vi "add overlays.vi"(8 "error in (no error)":errorcluster, 9 "location constraints":T2(array[cluster]), 10 "Overlay Rectangles":T1(array[cluster]), 11 "color ims":cluster{"xy im":T3, "xz im":T3, "zy im":T3}) -> (0 "error out":errorcluster, 3 "color ims out":cluster{"xy im":T3, "xz im":T3, "zy im":T3})   [LabVIEW 2010]
uses:
  <vilib>/vision/Image Controls.llb/IMAQ Image.ctl
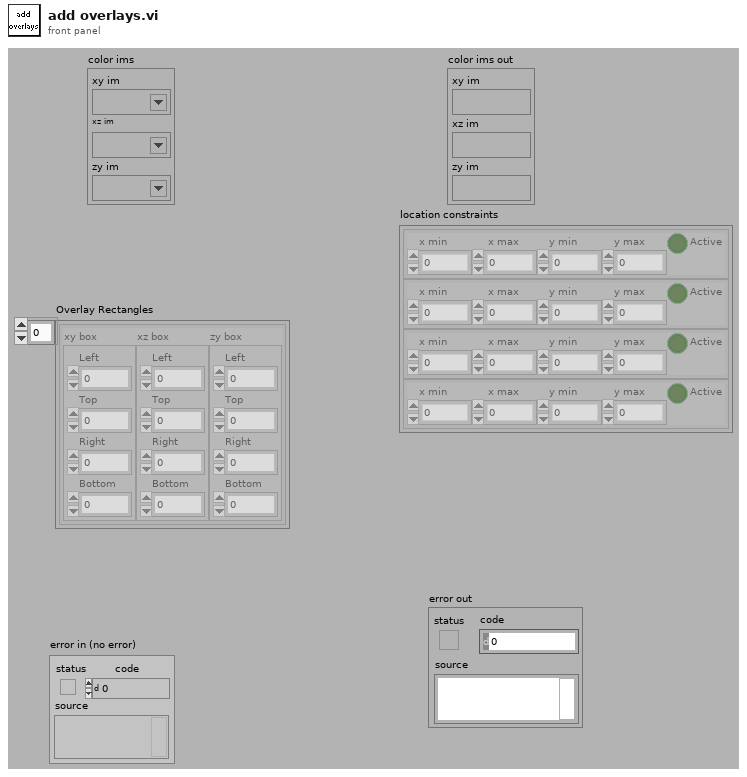
[diagram p1: front panel]
types:
  T1 = cluster{"xy box":cluster{"Left":i32, "Top":i32, "Right":i32, "Bottom":i32}, "xz box":cluster{"Left":i32, "Top":i32, "Right":i32, "Bottom":i32}, "zy box":cluster{"Left":i32, "Top":i32, "Right":i32, "Bottom":i32}}[]
  T2 = cluster{"x min":i32, "x max":i32, "y min":i32, "y max":i32, "Active":bool}[]
  T3 = typedef "IMAQ Image.ctl" = refnum<image>
  T4 = cluster{"Desired Font (Application)":enum16{"User-specified Font", "Application Font", "System Font", "Dialog Font"}, "[User-specified Font]":cluster{"Font Name":string, "Size":i16, "Strikeout?":bool, "Italic?":bool, "Underline?":bool, "Outline?":bool, "Shadow?":bool, "Bold?":bool, "Rotation Angle":dbl}, "Horizontal Alignment":i16, "Vertical Alignment":i16}
  T5 = cluster{"Left":i32, "Top":i32, "Right":i32, "Bottom":i32}
  T6 = cluster{"Left":i32, "Top":i32, "Right":i32, "Bottom":i32}[]
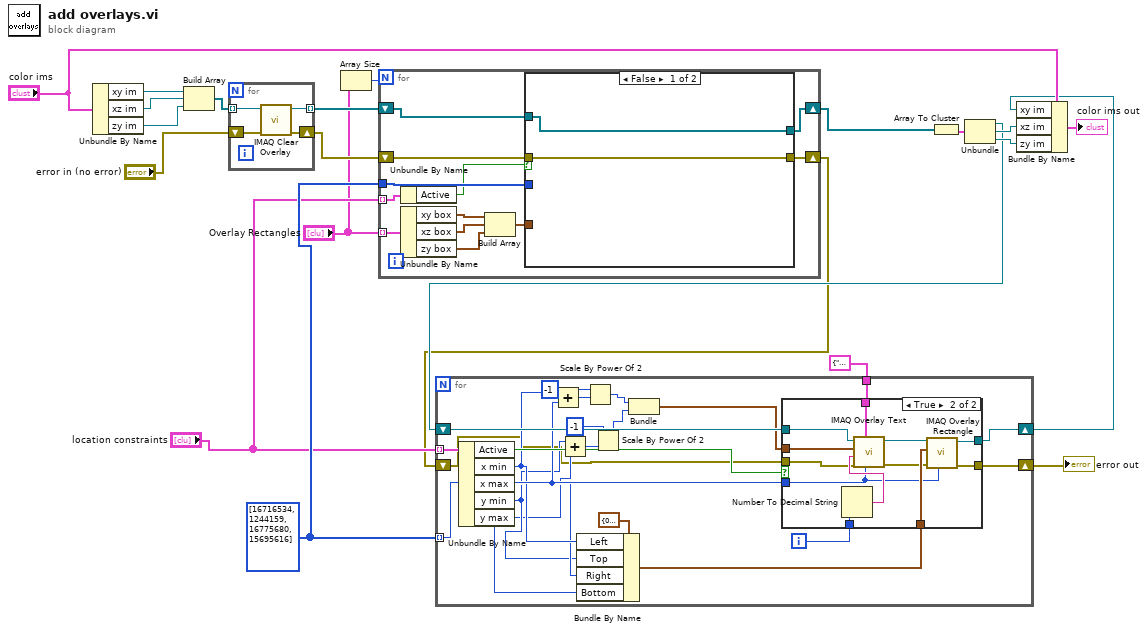
[diagram p0: block diagram]
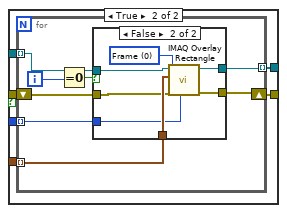
[diagram p2: hidden frame]
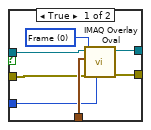
[diagram p3: hidden frame]
diagram:
  w10 = u32[] [16716534, 1244159, 16775680, 15695616]
  n1 = Unbundle By Name("color ims") -> ("xy im"=w22:T3, "xz im"=w21:T3, "zy im"=w20:T3)
  n2 = Build Array(w22, w21, w20) -> (w12:T3[])
  n3 = for {
    shift-right: [w25] -> w9
    shift-left: "error in (no error)" -> [w26]
    tunnel: w12 -> [w24] mode=indexing
    tunnel: [w23] -> w11 mode=indexing
    n4 = call "IMAQ Clear Overlay"("error in (no error)"=w26, "Image"=w24) -> ("error out"=w25:errorcluster, "Image Out"=w23:T3)  [unwired: 8 in]
  }
  n5 = Array Size(array="Overlay Rectangles") -> (size(s)=w2:i32)
  n6 = for {
    N: w2 -> [_]
    tunnel: "Overlay Rectangles" -> [w33] mode=indexing
    shift-right: [w29] -> w8
    shift-left: w11 -> [w32]
    tunnel: w10 -> [w31]
    shift-right: [w34] -> w3
    shift-left: w9 -> [w30]
    tunnel: "location constraints" -> [w28] mode=indexing
    n7 = Unbundle By Name(w28) -> ("Active"=w27:bool)
    n8 = Unbundle By Name(w33) -> ("xy box"=w38:T5, "xz box"=w37:T5, "zy box"=w36:T5)
    n9 = Build Array(w38, w37, w36) -> (w35:T6)
    n10 = case shown="False" w27 {
      tunnel: w35 -> [_ w46]
      tunnel: [w39 w45] -> w34
      tunnel: w32 -> [w40 w44]
      tunnel: w31 -> [_ w43]
      tunnel: w30 -> [w39 w42]
      tunnel: [w40 w41] -> w29
      frame False {
      }
      frame True {
        n11 = for {
          tunnel: w44 -> [w52] mode=indexing
          tunnel: w46 -> [w54] mode=indexing
          shift-right: [w49] -> w45
          shift-left: w42 -> [w50]
          tunnel: [w53] -> w41 mode=indexing
          tunnel: w43 -> [w51] mode=indexing
          i -> [w47]
          n12 = Equal To 0?(x=w47) -> (x = 0?=w48:bool)
          n13 = case shown="False" w48 {
            tunnel: w54 -> [w61 w68]
            tunnel: [w59 w66] -> w53
            tunnel: w52 -> [w58 w65]
            tunnel: w51 -> [w57 w64]
            tunnel: w50 -> [w56 w63]
            tunnel: [w55 w62] -> w49
            frame True {
              w60 = u32 0 items=["Frame", "Fill"] ("Drawing Mode (Frame)")
              n14 = call "IMAQ Overlay Oval"("Color"=w57, "error in (no error)"=w56, "Drawing Mode (Frame)"=w60, "Bounding Rectangle"=w61, "Image"=w58) -> ("error out"=w55:errorcluster, "Image Out"=w59:T3)  [unwired: 5 in]
            }
            frame False {
              w67 = u32 0 items=["Frame", "Fill"] ("Drawing Mode (Frame)")
              n15 = call "IMAQ Overlay Rectangle"("Color"=w64, "error in (no error)"=w63, "Drawing Mode (Frame)"=w67, "Rectangle"=w68, "Image"=w65) -> ("error out"=w62:errorcluster, "Image Out"=w66:T3)  [unwired: 5 in]
            }
          }
        }
      }
    }
  }
  n16 = Array To Cluster(array=w8) -> (cluster=w18:cluster{"[0]":T3, "[1]":T3, "[2]":T3})
  n17 = Unbundle(w18) -> ("[0]"=w6:T3, "[1]"=w17:T3, "[2]"=w16:T3)
  n18 = for {
    tunnel: "location constraints" -> [w86] mode=indexing
    tunnel: w10 -> [w90] mode=indexing
    shift-right: [w88] -> w5
    shift-left: w6 -> [w82]
    tunnel: T4 {"Desired Font (Application)"=enum."Application Font", "[User-specified Font]"={"Font Name"="", "Size"=12, "Strikeout?"=FALSE, "Italic?"=FALSE, "Underline?"=FALSE, "Outline?"=FALSE, "Shadow?"=FALSE, "Bold?"=FALSE, "Rotation Angle"=0.0}, "Horizontal Alignment"=1, "Vertical Alignment"=2} ("Font, Size & Style") -> [w87]
    shift-right: [w70] -> w4
    shift-left: w3 -> [w69]
    i -> [w89]
    n19 = Unbundle By Name(w86) -> ("Active"=w85:bool, "x min"=w81:i32, "x max"=w80:i32, "y min"=w79:i32, "y max"=w78:i32)
    n20 = Add(x=w81, y=w80) -> (x+y=w77:i32)
    n21 = Add(x=w79, y=w78) -> (x+y=w75:i32)
    n22 = Bundle By Name(cluster=T5 {"Left"=0, "Top"=0, "Right"=0, "Bottom"=0} ("Rectangle"), "Left"=w81, "Top"=w79, "Right"=w80, "Bottom"=w78) -> (w83:T5)
    n23 = Scale By Power Of 2(n=-1, x=w77) -> (x*2^n=w73:i32)
    n24 = Scale By Power Of 2(n=-1, x=w75) -> (x*2^n=w72:i32)
    n25 = Bundle(w73, w72) -> (w71:cluster{i32, i32})  [unwired: 1 in]
    n26 = case shown="True" w85 {
      tunnel: w90 -> [_ w98]
      tunnel: w89 -> [_ w103]
      tunnel: [w92 w97] -> w88
      tunnel: w87 -> [_ w102]
      tunnel: w83 -> [_ w100]
      tunnel: w82 -> [w92 w96]
      tunnel: w71 -> [_ w95]
      tunnel: [w91 w94] -> w70
      tunnel: w69 -> [w91 w93]
      frame False {
      }
      frame True {
        n27 = Number To Decimal String(number=w103) -> (decimal integer string=w104:string)  [unwired: 1 in]
        n28 = call "IMAQ Overlay Text"("Text Color (black)"=w98, "Font, Size & Style"=w102, "error in (no error)"=w93, "String"=w104, "Origin"=w95, "Image"=w96) -> ("error out"=w99:errorcluster, "Image Out"=w101:T3)  [unwired: 4 in]
        n29 = call "IMAQ Overlay Rectangle"("Color"=w98, "error in (no error)"=w99, "Rectangle"=w100, "Image"=w101) -> ("error out"=w94:errorcluster, "Image Out"=w97:T3)  [unwired: 6 in]
      }
    }
  }
  "error out" <- w4
  n30 = Bundle By Name(cluster="color ims", "xy im"=w5, "xz im"=w17, "zy im"=w16) -> (→"color ims out":cluster{"xy im":T3, "xz im":T3, "zy im":T3})
